vi "ODE-VI-28032016.vi"(0 "Param_Value":dbl[](array[numeric])=[0.35, 180.0, 0.3], 1 "Mod_Value":dbl[](array[numeric]), 3 "Param_IDs":string[](array[string])=["k1", "k2", "compartment"], 4 "Mod_IDs":string[](array[string]), 5 "Initial Conditions for  variables":dbl[](array[numeric])=[0.00015, 0.0], 6 "Simulation Parameters":T2={"Initial Time"=0.1, "Final Time"=1e-07, "Time Step"=0.0001, "Absolute Tolerance"=0.0, "Relative Tolerance"=1.0, "Type of Continuous Solver"=enum."Runge-Kutta 1 (Euler)", "Discrete Time Step"=1.0, "Minimum Time Step"=0.1, "Maximum Time Step"=0.0, "Initial Time Step"=10.0} {"Initial Time Step" min=0.0; "Maximum Time Step" min=0.0; "Minimum Time Step" min=0.0; "Discrete Time Step" min=0.0; "Relative Tolerance" min=0.0; "Absolute Tolerance" min=0.0; "Time Step" min=0.0}, 7 "ODE Right Hand Side":string[](array[string])=["-(compartment*k1*a0)+(compartment*k2*a1^2)", "-2*(compartment*k2*a1^2)+2*(compartment*k1*a0)"], 8 "Rest_Sp_IDs":string[](array[string]), 9 "Del Events":bool, 10 "Event Info":T1, 11 "X (name of variables)":string[](array[string])=["a0", "a1"], 12 "All Variables":string[](array[string]), 13 "Rest_Sp_Init_Amnt":string[](array[string])) -> (14 "Concentration vs. Time":cluster{"times":dbl[], dbl[]}[](graph), 16 "Mod_IDs Out":string[](array[string]), 17 "Rest_Sp_IDs Out":string[](array[string]), 19 "Sim Data":cluster{"times":dbl[], "outputs":dbl[][]} {"outputs" format="%#.9g"})   [LabVIEW 2014]
doc: "This example demonstrates how to use the polymorphic ODE solver in both Formula Sting mode and VI mode. Note that VI mode allows the user to set the values of constants via front panel controls, and the formula is implemented as a call by reference to another VI."
uses:
  ODE Simulation Parameters.ctl
  <vilib>/Simulation/Implementation/Shared/SIM Continuous Solvers.ctl
  Event Info.ctl
  Stop ODE.vi
  <vilib>/gmath/ode.llb/ODE Solver formula string.vi
  Sim status.vi
  <vilib>/gmath/NI_Gmath.lvlib
panel:
  out "error out":errorcluster
  out "subarray 2":dbl[](array[numeric])
  out "Array":dbl[][](array[numeric])
  out "transposed array":dbl[][](array[numeric])
  out "Assign Val":string[][](array[string])
  out "Assign Var Idx":i32[][](array[numeric])
  out "Var Idx":i32[](array[numeric])
  out "Math Val":string[](array[string])
  out "Math Op":string[](array[string])
  out "outputs":dbl[][](array[numeric])
  out "subarray":dbl[][](array[numeric])
  out "Flag":i32[](array[numeric])
  out "Delay Val Tot":dbl[](array[numeric])
  out "Delay Val":dbl[](array[numeric])
  out "Delay Val":dbl
  out "Priority":dbl[](array[numeric])
  out "Event Idx":i32
  out "Delay":dbl[](array[numeric])
  out "Total Mods":i32
  out "Time":dbl[](array[numeric])
  out "current data size":i32[](array[numeric])
  # "%"
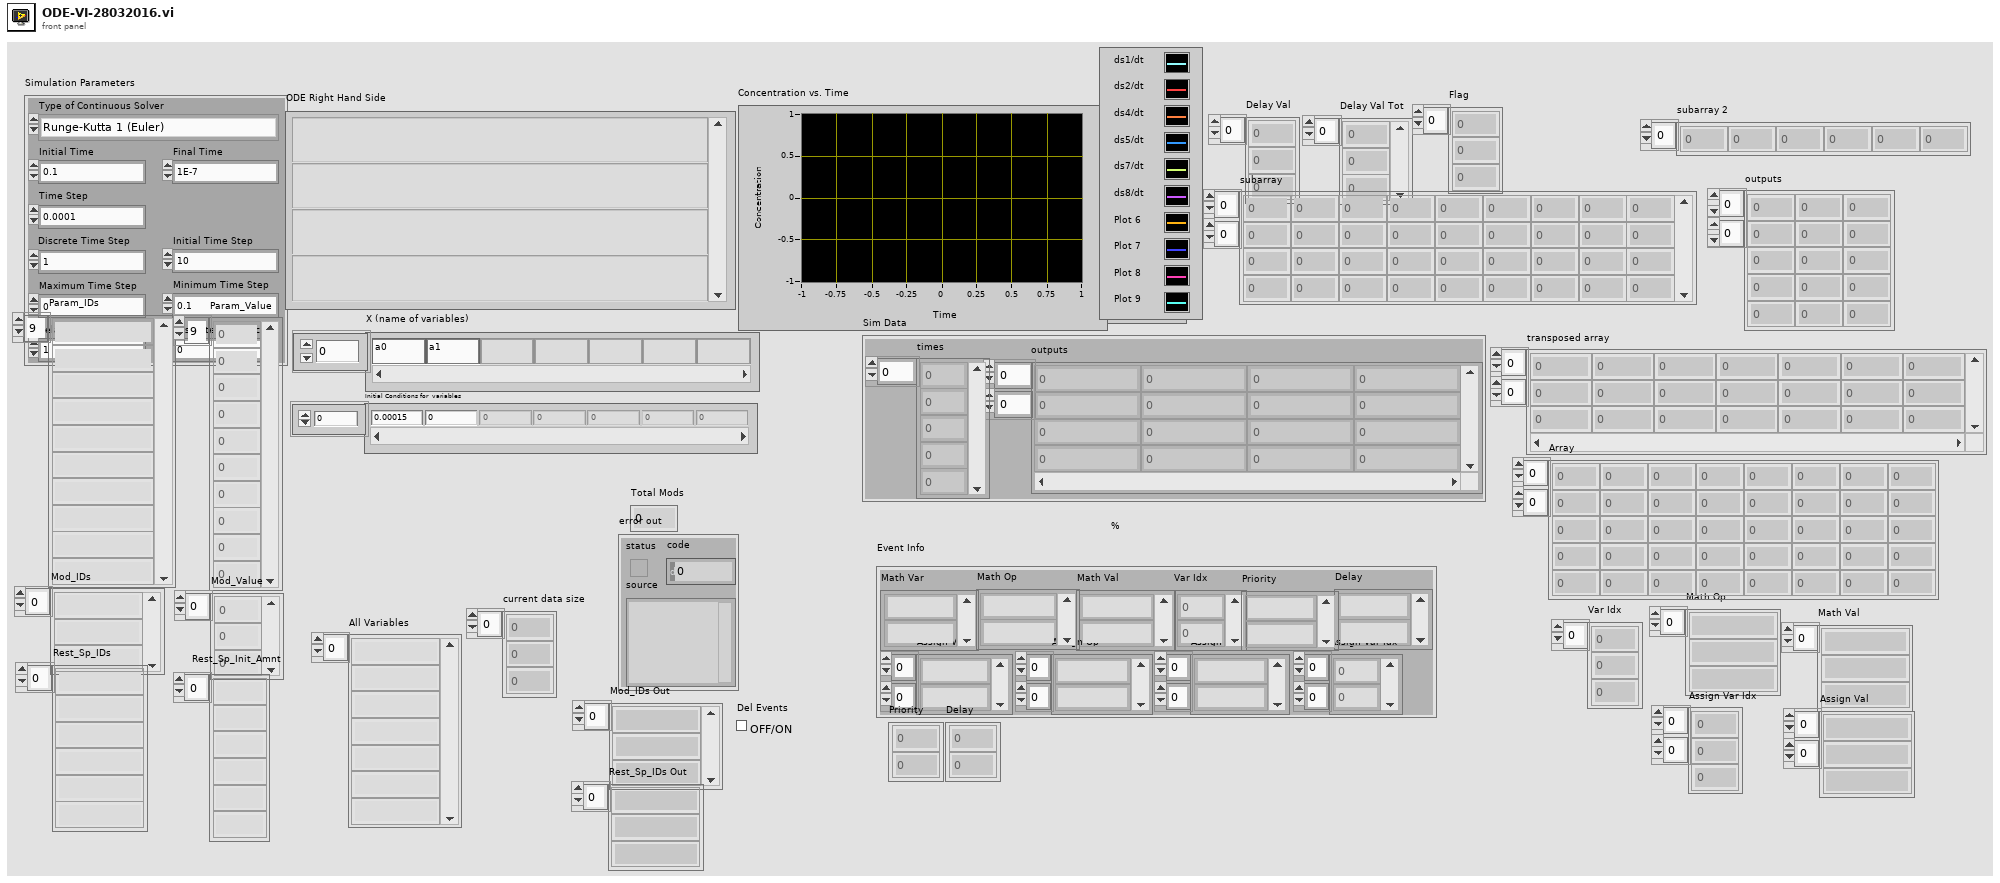
[diagram p1: front panel]
types:
  T1 = typedef "Event Info.ctl" = cluster{"Math Var":string[], "Math Op":string[], "Math Val":string[], "Assign Var":string[][], "Assign Op":string[][], "Assign Val":string[][], "Var Idx":i32[], "Assign Var Idx":i32[][], "Delay":string[], "Priority":string[]}
  T2 = typedef "ODE Simulation Parameters.ctl" = cluster{"Initial Time":dbl, "Final Time":dbl, "Time Step":dbl, "Absolute Tolerance":dbl, "Relative Tolerance":dbl, "Type of Continuous Solver":T3, "Discrete Time Step":dbl, "Minimum Time Step":dbl, "Maximum Time Step":dbl, "Initial Time Step":dbl}
  T3 = typedef "SIM Continuous Solvers.ctl" = enum16{"Runge-Kutta 1 (Euler)", "Runge-Kutta 2", "Runge-Kutta 3", "Runge-Kutta 4", "Runge-Kutta 23 (variable)", "Runge-Kutta 45 (variable)", "BDF (variable)", "Adams-Moulton (variable)", "Rosenbrock (variable)", "Discrete States Only"}
  T4 = cluster{"ODE Right Hand Side":string[], "X (name of variables)":string[], "time":string}
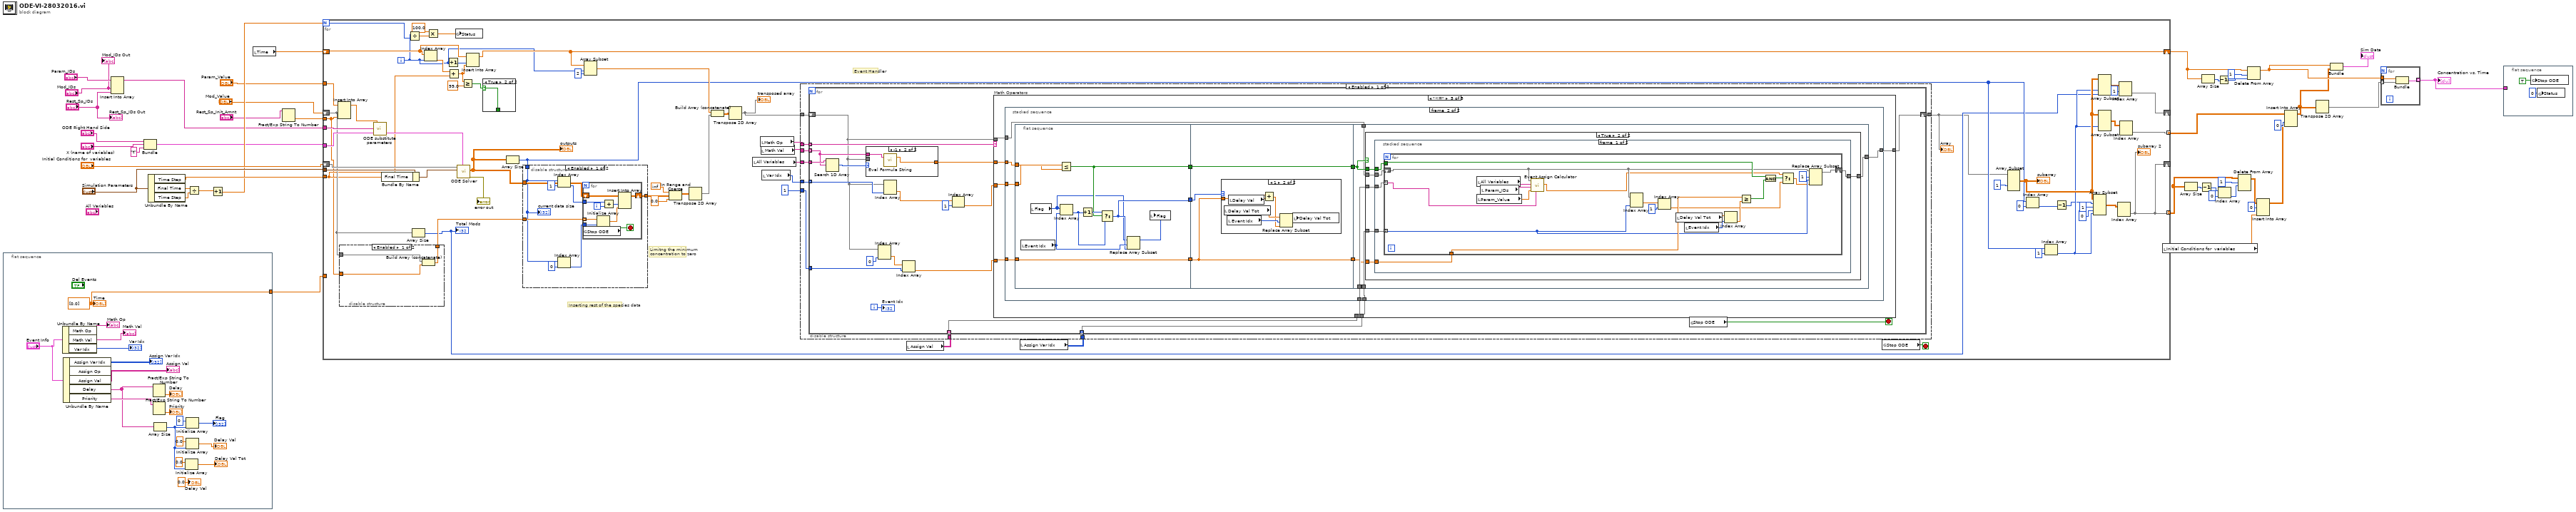
[diagram p0: block diagram]
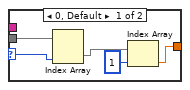
[diagram p5: hidden frame]
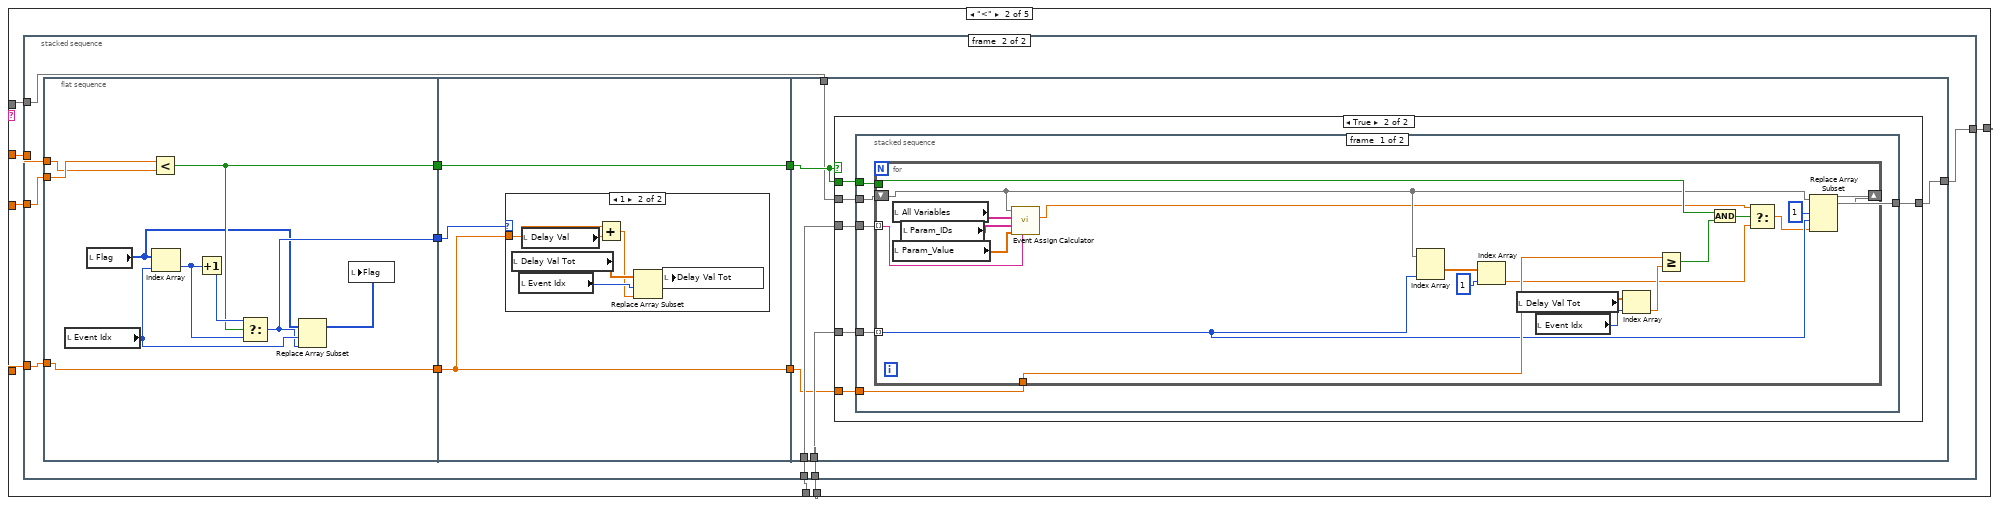
[diagram p7: hidden frame]
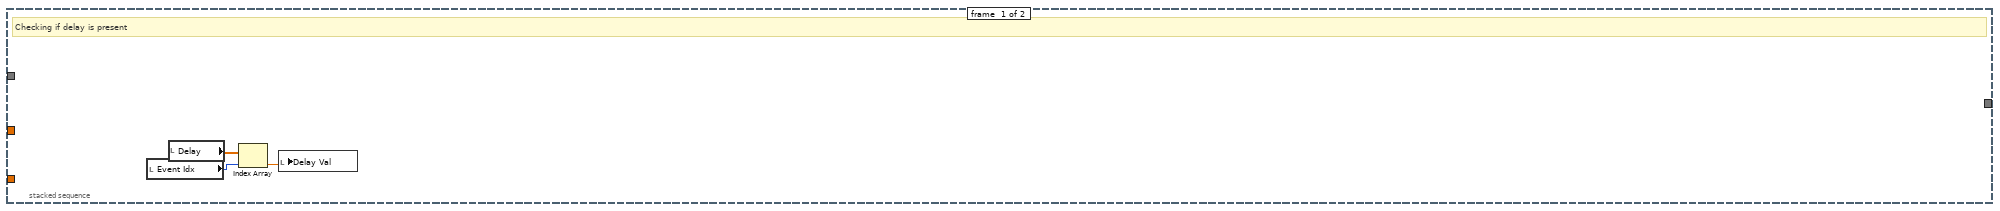
[diagram p8: hidden frame]
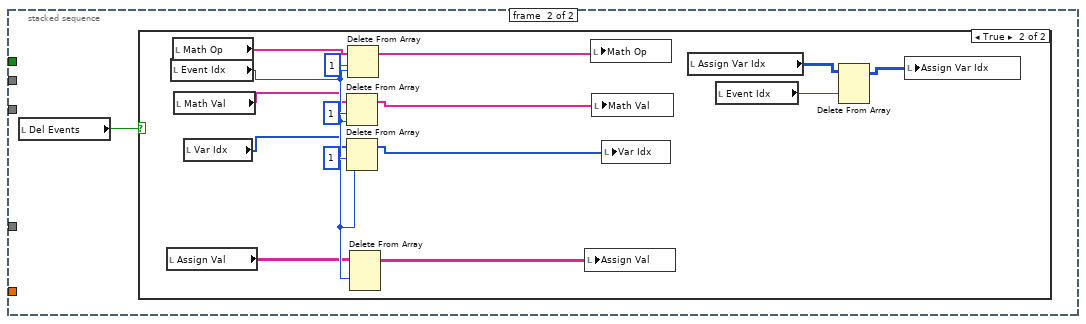
[diagram p11: hidden frame]
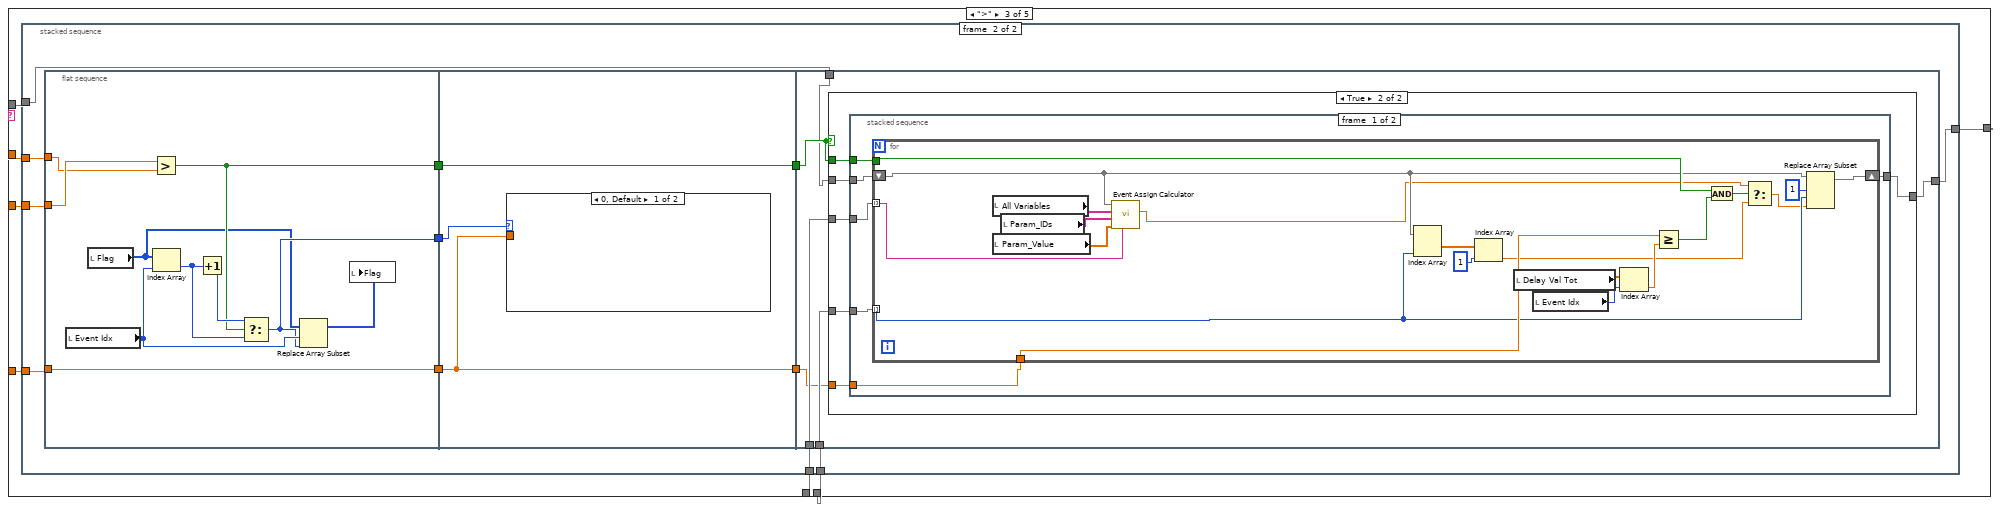
[diagram p13: hidden frame]
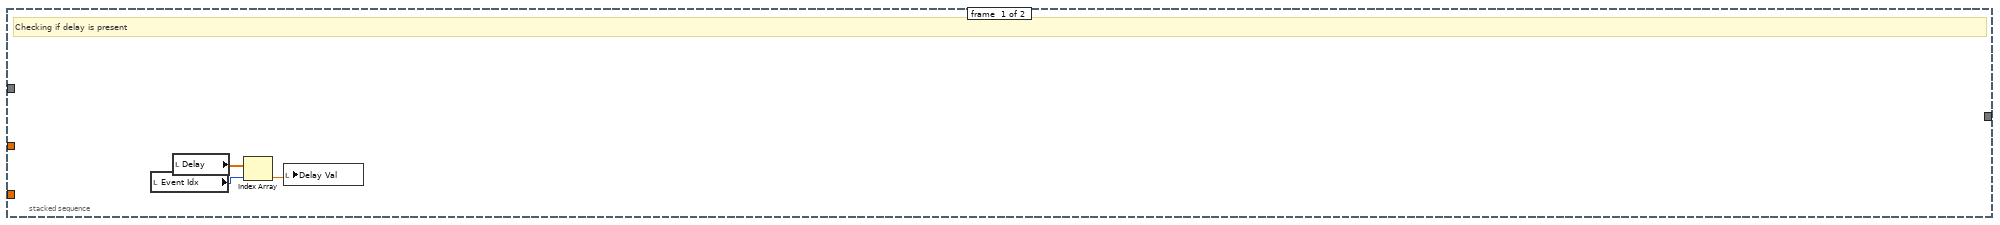
[diagram p14: hidden frame]
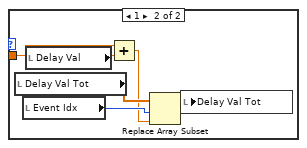
[diagram p15: hidden frame]
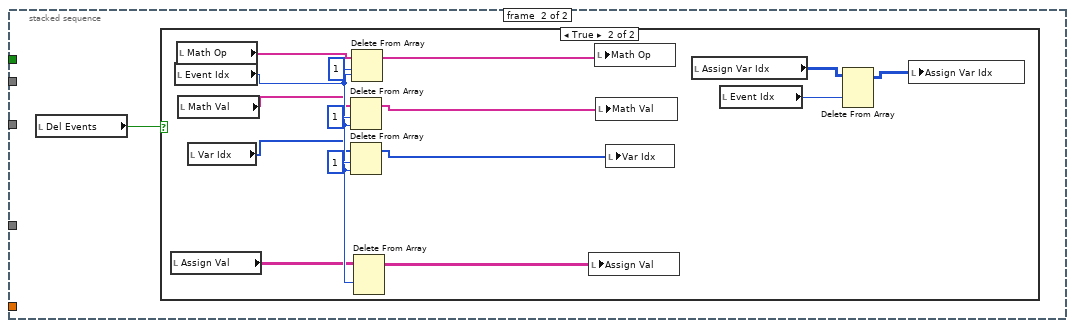
[diagram p17: hidden frame]
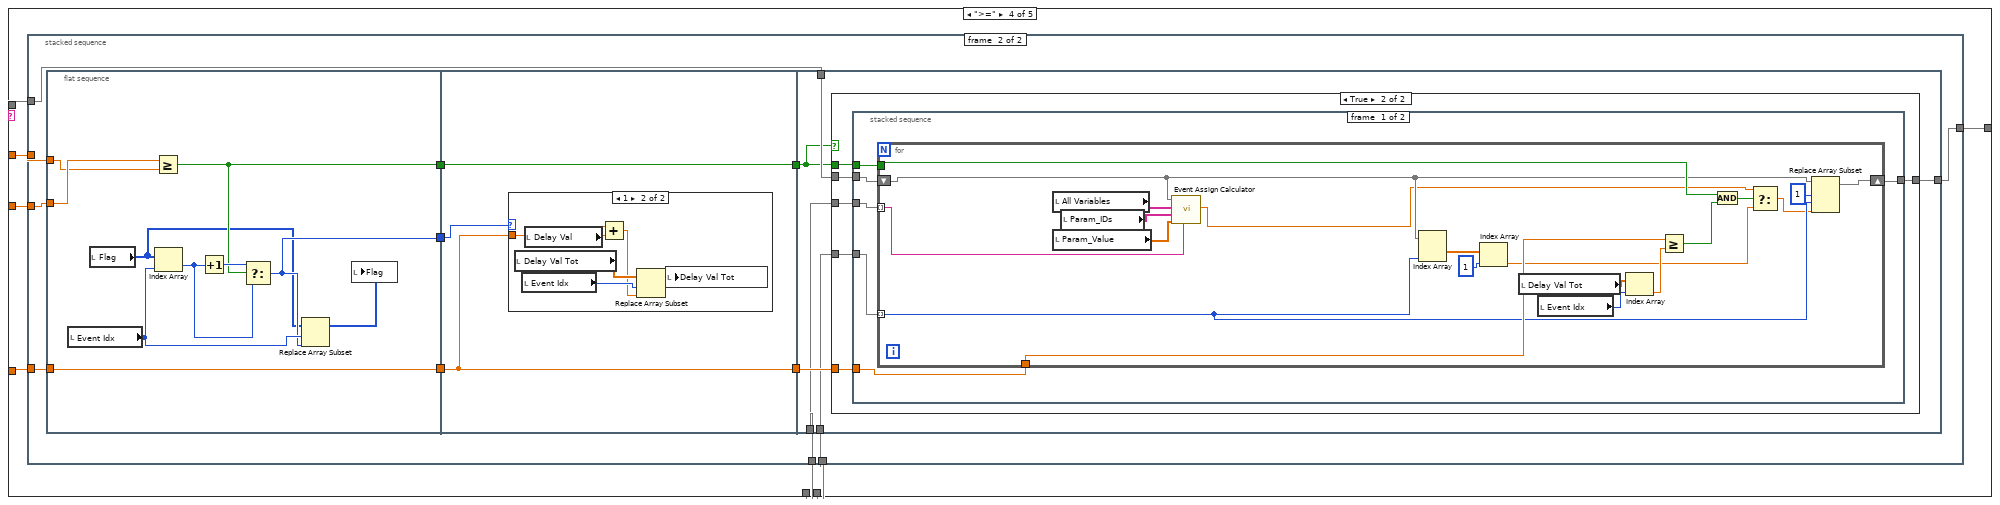
[diagram p19: hidden frame]
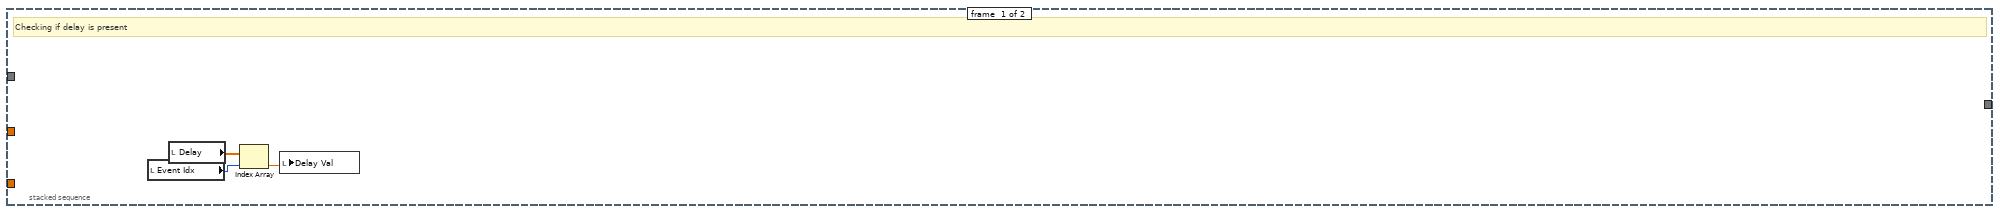
[diagram p20: hidden frame]
diagram:
  n1 = flat-sequence {
    tunnel: [w43] -> w4
    frame #0 {
      w43 = dbl[] [0.0]
      n2 = Unbundle By Name("Event Info") -> ("Math Op"=→"Math Op":string[], "Math Val"=→"Math Val":string[], "Var Idx"=→"Var Idx":i32[])
      n3 = Unbundle By Name("Event Info") -> ("Assign Var Idx"=→"Assign Var Idx":i32[][], "Assign Val"=→"Assign Val":string[][], "Delay"=w52:string[], "Priority"=w55:string[])  [unwired: 1 out]
      n4 = Fract/Exp String To Number(string=w52) -> (number=→"Delay":dbl[])  [unwired: 3 in, 1 out]
      n5 = Fract/Exp String To Number(string=w55) -> (number=→"Priority":dbl[])  [unwired: 3 in, 1 out]
      n6 = Array Size(array=w52) -> (size(s)=w47:i32)
      n7 = Initialize Array(0.0 ("element"), w47) -> (→"Delay Val Tot":dbl[])
      n8 = Initialize Array(0 ("element"), w47) -> (→"Flag":i32[])
      n9 = Initialize Array(0.0 ("element"), w47) -> (→"Delay Val":dbl[])
      "Time" <- w43
      "Delay Val" <- 0.0 ("Delay Val")
    }
  }
  n10 = Insert Into Array(array="Param_IDs", new element #1="Mod_IDs", new element #2="Rest_Sp_IDs") -> (w8:string[])  [unwired: 1 in]
  n11 = Bundle("ODE Right Hand Side"="ODE Right Hand Side", "X (name of variables)"="X (name of variables)", "time"="t") -> (w9:T4)  [unwired: 1 in]
  n12 = Unbundle By Name("Simulation Parameters") -> ("Time Step"=w33:dbl, "Final Time"=w35:dbl, "Time Step"=w34:dbl)
  n13 = Divide(x=w35, y=w34) -> (x/y=w31:dbl)
  n14 = Increment(x=w31) -> (x+1=w30:dbl)
  n15 = local read "Time"() -> (w32:dbl[])
  n16 = Fract/Exp String To Number(string="Rest_Sp_Init_Amnt") -> (number=w1:dbl[])  [unwired: 3 in, 1 out]
  n17 = for {
    N: w30 -> [w77]
    tunnel: "Simulation Parameters" -> [w108]
    shift-right: [w67] -> _
    shift-left: "Initial Conditions for  variables" -> [w123]
    shift-right: [w106] -> w28
    shift-left: w32 -> [w110]
    tunnel: [w67] -> w12 mode=indexing
    tunnel: w33 -> [w87]
    tunnel: [w101] -> w13 mode=indexing
    tunnel: w9 -> [w99]
    tunnel: w8 -> [w98]
    tunnel: "Param_Value" -> [w97]
    shift-right: [w80] -> _
    shift-left: "Mod_Value" -> [w93]
    tunnel: w4 -> [_]
    tunnel: w1 -> [w62]
    i -> [w78]
    stop <- w91 stop-if-true
    # "Event Handler"
    # "Limitng the minimum \nconcentration to zero"
    # "Inserting rest of the species data"
    n18 = Insert Into Array(array=w97, new element #1=w93, new element #2=w62) -> (w96:dbl[])  [unwired: 1 in]
    n19 = disable-structure shown="Enabled" {
      disable-tunnel: [w126 _] -> w121
      disable-tunnel: w93 -> [w125 _]
      disable-tunnel: w62 -> [w124 _]
      frame Enabled {
        n20 = Build Array (concatenate)(w125, w124) -> (w126:dbl[])
      }
      frame Disabled {
      }
    }
    n21 = call "ODE substitute parameters.vi"("Formula String Parameters"=w99, "parameters"=w98, "values"=w96) -> ("Formula String Parameters with substitutions"=w100:T4)  [unwired: 2 out]
    n22 = Bundle By Name(cluster=w108, "Final Time"=w87) -> (w107:T2)
    n23 = Divide(x=w78, y=w77) -> (x/y=w76:dbl)
    n24 = Array Size(array=w93) -> (size(s)=w92:i32)
    "Total Mods" <- w92
    n25 = Index Array(array=w110, index=w78) -> (element=w111:dbl)
    n26 = Multiply(x=100.0, y=w76) -> (x*y=w74:dbl)
    n27 = Increment(x=w78) -> (x+1=w109:i32)
    n28 = Add(x=w111, y=w87) -> (x+y=w84:dbl)
    n29 = global write "Sim status.vi" "Status"(w74) -> ()
    n30 = call-poly <vilib>:"ODE Solver.vi"("ODE RHS"=w100, "simulation parameters"=w107, "x0"=w123) -> ("error out"=→"error out":errorcluster, "outputs"=w122:dbl[][])  [unwired: 3 in, 4 out]
    "outputs" <- w122
    n31 = Greater Or Equal?(x=w84, y=99.0) -> (x >= y?=w82:bool)
    n32 = Insert Into Array(array=w110, index=w109, new element=w84) -> (w106:dbl[])
    n33 = case shown="True" w82 {
      selector: w82 -> [w145 w146]
      tunnel: [w145 w146] -> _
      frame False {
      }
      frame True {
      }
    }
    n34 = Array Size(array=w122) -> (size(s)=w103:i32[])
    n35 = disable-structure shown="Enabled" {
      disable-tunnel: w122 -> [w130 w144]
      disable-tunnel: w121 -> [w129 _]
      disable-tunnel: [w128 w144] -> w118
      disable-tunnel: w103 -> [w127 _]
      frame Enabled {
        n36 = Index Array(array=w127, index=1) -> (element=w133:i32)
        n37 = Index Array(array=w127, index=0) -> (element=w131:i32)
        n38 = for {
          tunnel: w129 -> [w140] mode=indexing
          tunnel: w133 -> [w142]
          tunnel: w131 -> [w139]
          shift-right: [w136] -> w128
          shift-left: w130 -> [w137]
          i -> [w143]
          stop <- w135 stop-if-true
          n39 = global read "Stop ODE.vi" "Stop ODE"() -> (w135:bool)
          n40 = Initialize Array(w140, w139) -> (w138:dbl[])
          n41 = Add(x=w142, y=w143) -> (x+y=w141:i32)
          n42 = Insert Into Array(array=w137, index (col)=w141, new element=w138) -> (w136:dbl[][])  [unwired: 1 in]
        }
        "current data size" <- w127
      }
      frame Disabled {
      }
    }
    n43 = Array Subset(array=w106, index=w78, length=2) -> (w104:dbl[])
    n44 = In Range and Coerce(upper limit=inf, x=w118, lower limit=0.0) -> (coerced(x)=w89:dbl[][])  [unwired: 1 out]
    n45 = Transpose 2D Array(2D array=w89) -> (transposed array=w88:dbl[][])
    n46 = Build Array (concatenate)(w104, w88) -> (w90:dbl[][])
    n47 = Transpose 2D Array(2D array=w90) -> (transposed array=w86:dbl[][])
    "transposed array" <- w86
    n48 = local read "All Variables"() -> (w68:string[])
    n49 = local read "Math Op"() -> (w73:string[])
    n50 = local read "Math Val"() -> (w72:string[])
    n51 = local read "Var Idx"() -> (w71:i32[])
    n52 = local read "Assign Val"() -> (w69:string[][])
    n53 = local read "Assign Var Idx"() -> (w70:i32[][])
    n54 = disable-structure shown="Enabled" {
      disable-tunnel: w73 -> [w155 w576]
      disable-tunnel: w72 -> [w154 w577]
      disable-tunnel: w71 -> [w153 w578]
      disable-tunnel: w69 -> [w148 w575]
      disable-tunnel: w70 -> [w152 w574]
      disable-tunnel: [w151 w580] -> w66
      disable-tunnel: w86 -> [w150 w581]
      disable-tunnel: 1 ("index") -> [w149 w579]
      disable-tunnel: w68 -> [w147 _]
      frame Enabled {
        n55 = for {
          tunnel: w155 -> [w174] mode=indexing
          tunnel: w154 -> [w158] mode=indexing
          tunnel: w153 -> [w173] mode=indexing
          tunnel: w148 -> [w169] mode=indexing
          tunnel: w152 -> [w172] mode=indexing
          shift-right: [w167] -> w151
          shift-left: w150 -> [w156]
          tunnel: w149 -> [w161]
          tunnel: w147 -> [w159]
          i -> [w170]
          stop <- w171 stop-if-true
          n56 = Search 1D Array(1D array=w159, element=w158) -> (index of element=w157:i32)  [unwired: 1 in]
          n57 = case shown="-1" w157 {
            selector: w157 -> [w178 _]
            tunnel: [w175 w180] -> w168
            tunnel: w158 -> [_ w181]
            tunnel: w156 -> [w179 _]
            frame 0, Default {
              n58 = Index Array(array=w179, index (col)=w178) -> (element=w176:dbl[])  [unwired: 1 in]
              n59 = Index Array(array=w176, index=1) -> (element=w175:dbl)
            }
            frame -1 {
              n60 = call <vilib>:"Eval Formula String.vi"("formula"=w181) -> ("y value"=w180:dbl)  [unwired: 1 in, 1 out]
            }
          }
          n61 = Index Array(array=w156, index (col)=0 ("disabled index (col)")) -> (element=w162:dbl[])  [unwired: 1 in]
          n62 = Index Array(array=w156, index (col)=w173) -> (element=w165:dbl[])  [unwired: 1 in]
          n63 = Index Array(array=w162, index=w161) -> (element=w160:dbl)
          n64 = Index Array(array=w165, index=1) -> (element=w164:dbl)
          n65 = case "Math Operators" shown="\"<=\"" w174 {
            tunnel: w168 -> [_ w188 w284 w380 w476]
            tunnel: [w182 w187 w283 w379 w475] -> w167
            tunnel: w156 -> [w182 w189 w285 w381 w477]
            tunnel: w169 -> [_ w186 w282 w378 w474]
            tunnel: w172 -> [_ w185 w281 w377 w473]
            tunnel: w164 -> [_ w184 w280 w375 w472]
            tunnel: w160 -> [_ w183 w279 w376 w471]
            frame "False", Default {
            }
            frame "<" {
              n66 = stacked-sequence {
                tunnel: w188 -> [_ w204]
                tunnel: w189 -> [_ w196]
                tunnel: [_ w195] -> w187
                tunnel: w186 -> [_ w198]
                tunnel: w185 -> [_ w197]
                tunnel: w184 -> [_ w194]
                tunnel: w183 -> [_ w193]
                frame #0 {
                  # "Checking if delay is present"
                  n67 = local read "Event Idx"() -> (w191:i32)
                  n68 = local read "Delay"() -> (w192:dbl[])
                  n69 = Index Array(array=w192, index=w191) -> (element=w190:dbl)
                  n70 = local write "Delay Val"(w190) -> ()
                }
                frame #1 {
                  n71 = flat-sequence {
                    tunnel: w194 -> [w214]
                    tunnel: w204 -> [w213]
                    tunnel: [w208] -> w203
                    tunnel: [w207] -> w202
                    tunnel: [w205] -> w201
                    tunnel: w193 -> [w205]
                    tunnel: w203 -> [w216]
                    tunnel: w202 -> [w217]
                    tunnel: w201 -> [w215]
                    tunnel: [w217] -> w200
                    tunnel: [w215] -> w199
                    tunnel: w200 -> [w229]
                    tunnel: w199 -> [w225]
                    tunnel: w196 -> [w228]
                    tunnel: w197 -> [w226]
                    tunnel: w198 -> [w227]
                    tunnel: [w224] -> w195
                    frame #0 {
                      n72 = local read "Event Idx"() -> (w211:i32)
                      n73 = local read "Flag"() -> (w206:i32[])
                      n74 = Less?(x=w214, y=w213) -> (x < y?=w207:bool)
                      n75 = Index Array(array=w206, index=w211) -> (element=w210:i32)
                      n76 = Increment(x=w210) -> (x+1=w209:i32)
                      n77 = Select(t=w209, s=w207, f=w210) -> (s? t:f=w208:i32)
                      n78 = Replace Array Subset(array=w206, new element=w208, index=w211) -> (w212:i32[])
                      n79 = local write "Flag"(w212) -> ()
                    }
                    frame #1 {
                      n80 = case shown="1" w216 {
                        tunnel: w215 -> [_ w222]
                        frame 0, Default {
                        }
                        frame 1 {
                          n81 = local read "Delay Val Tot"() -> (w221:dbl[])
                          n82 = local read "Event Idx"() -> (w219:i32)
                          n83 = local read "Delay Val"() -> (w223:dbl)
                          n84 = Add(x=w222, y=w223) -> (x+y=w218:dbl)
                          n85 = Replace Array Subset(array=w221, new element=w218, index=w219) -> (w220:dbl[])
                          n86 = local write "Delay Val Tot"(w220) -> ()
                        }
                      }
                    }
                    frame #2 {
                      n87 = case shown="True" w229 {
                        tunnel: w229 -> [_ w236]
                        tunnel: w225 -> [_ w235]
                        tunnel: w228 -> [w230 w234]
                        tunnel: w226 -> [_ w233]
                        tunnel: w227 -> [_ w232]
                        tunnel: [w230 w231] -> w224
                        frame False {
                        }
                        frame True {
                          n88 = stacked-sequence {
                            tunnel: w236 -> [w242 _]
                            tunnel: w235 -> [w241 _]
                            tunnel: w234 -> [w240 _]
                            tunnel: w233 -> [w239 _]
                            tunnel: w232 -> [w238 _]
                            tunnel: [w237 _] -> w231
                            frame #0 {
                              n89 = for {
                                tunnel: w242 -> [w260]
                                tunnel: w241 -> [w259]
                                tunnel: w239 -> [w251] mode=indexing
                                tunnel: w238 -> [w244] mode=indexing
                                shift-right: [w249] -> w237
                                shift-left: w240 -> [w248]
                                n90 = local read "All Variables"() -> (w247:string[])
                                n91 = local read "Param_Value"() -> (w245:dbl[])
                                n92 = local read "Param_IDs"() -> (w246:string[])
                                n93 = call "Event Assign Calculator.vi"("Assign Val"=w244, "Param_Value"=w245, "Param_IDs"=w246, "All Variables"=w247, "transposed array"=w248) -> ("y value"=w243:dbl)  [unwired: 6 in]
                                n94 = Index Array(array=w248, index (col)=w251) -> (element=w254:dbl[])  [unwired: 1 in]
                                n95 = Index Array(array=w254, index=1) -> (element=w253:dbl)
                                n96 = local read "Delay Val Tot"() -> (w258:dbl[])
                                n97 = local read "Event Idx"() -> (w257:i32)
                                n98 = Index Array(array=w258, index=w257) -> (element=w256:dbl)
                                n99 = Greater Or Equal?(x=w259, y=w256) -> (x >= y?=w261:bool)
                                n100 = And(x=w260, y=w261) -> (x .and. y?=w262:bool)
                                n101 = Select(t=w243, s=w262, f=w253) -> (s? t:f=w250:dbl)
                                n102 = Replace Array Subset(array=w248, new element=w250, index (row)=1, index (col)=w251) -> (w249:dbl[][])
                              }
                            }
                            frame #1 {
                              n103 = local read "Del Events"() -> (w263:bool)
                              n104 = case shown="True" w263 {
                                frame False {
                                }
                                frame True {
                                n105 = local read "Assign Val"() -> (w268:string[][])
                                n106 = local read "Event Idx"() -> (w275:i32)
                                n107 = local read "Math Op"() -> (w274:string[])
                                n108 = local read "Math Val"() -> (w273:string[])
                                n109 = local read "Var Idx"() -> (w272:i32[])
                                n110 = Delete From Array(array=w273, length=1, index=w275) -> (array with subset deleted=w270:string[])  [unwired: 1 out]
                                n111 = Delete From Array(array=w272, length=1, index=w275) -> (array with subset deleted=w269:i32[])  [unwired: 1 out]
                                n112 = Delete From Array(array=w274, length=1, index=w275) -> (array with subset deleted=w271:string[])  [unwired: 1 out]
                                n113 = Delete From Array(array=w268, index (row)=w275) -> (array with subset deleted=w267:string[][])  [unwired: 2 in, 1 out]
                                n114 = local write "Assign Val"(w267) -> ()
                                n115 = local write "Math Op"(w271) -> ()
                                n116 = local write "Math Val"(w270) -> ()
                                n117 = local write "Var Idx"(w269) -> ()
                                n118 = local read "Assign Var Idx"() -> (w266:i32[][])
                                n119 = local read "Event Idx"() -> (w265:i32)
                                n120 = Delete From Array(array=w266, index (row)=w265) -> (array with subset deleted=w264:i32[][])  [unwired: 2 in, 1 out]
                                n121 = local write "Assign Var Idx"(w264) -> ()
                                }
                              }
                            }
                          }
                        }
                      }
                    }
                  }
                }
              }
            }
            frame ">" {
              n122 = stacked-sequence {
                tunnel: w284 -> [_ w300]
                tunnel: w285 -> [_ w292]
                tunnel: [_ w291] -> w283
                tunnel: w282 -> [_ w294]
                tunnel: w281 -> [_ w293]
                tunnel: w280 -> [_ w290]
                tunnel: w279 -> [_ w289]
                frame #0 {
                  # "Checking if delay is present"
                  n123 = local read "Event Idx"() -> (w287:i32)
                  n124 = local read "Delay"() -> (w288:dbl[])
                  n125 = Index Array(array=w288, index=w287) -> (element=w286:dbl)
                  n126 = local write "Delay Val"(w286) -> ()
                }
                frame #1 {
                  n127 = flat-sequence {
                    tunnel: w290 -> [w310]
                    tunnel: w300 -> [w309]
                    tunnel: w289 -> [w308]
                    tunnel: [w303] -> w299
                    tunnel: [w302] -> w298
                    tunnel: [w308] -> w297
                    tunnel: w299 -> [w312]
                    tunnel: w298 -> [w313]
                    tunnel: w297 -> [w311]
                    tunnel: [w313] -> w296
                    tunnel: [w311] -> w295
                    tunnel: w296 -> [w325]
                    tunnel: w295 -> [w321]
                    tunnel: w292 -> [w324]
                    tunnel: w293 -> [w322]
                    tunnel: w294 -> [w323]
                    tunnel: [w320] -> w291
                    frame #0 {
                      n128 = local read "Event Idx"() -> (w306:i32)
                      n129 = local read "Flag"() -> (w301:i32[])
                      n130 = Greater?(x=w310, y=w309) -> (0:w302:bool)
                      n131 = Index Array(array=w301, index=w306) -> (element=w305:i32)
                      n132 = Increment(x=w305) -> (x+1=w304:i32)
                      n133 = Select(t=w304, s=w302, f=w305) -> (s? t:f=w303:i32)
                      n134 = Replace Array Subset(array=w301, new element=w303, index=w306) -> (w307:i32[])
                      n135 = local write "Flag"(w307) -> ()
                    }
                    frame #1 {
                      n136 = case shown="0, Default" w312 {
                        tunnel: w311 -> [_ w318]
                        frame 0, Default {
                        }
                        frame 1 {
                          n137 = local read "Delay Val Tot"() -> (w317:dbl[])
                          n138 = local read "Event Idx"() -> (w315:i32)
                          n139 = local read "Delay Val"() -> (w319:dbl)
                          n140 = Add(x=w318, y=w319) -> (x+y=w314:dbl)
                          n141 = Replace Array Subset(array=w317, new element=w314, index=w315) -> (w316:dbl[])
                          n142 = local write "Delay Val Tot"(w316) -> ()
                        }
                      }
                    }
                    frame #2 {
                      n143 = case shown="True" w325 {
                        tunnel: w325 -> [_ w332]
                        tunnel: w321 -> [_ w331]
                        tunnel: w324 -> [w326 w330]
                        tunnel: w322 -> [_ w329]
                        tunnel: w323 -> [_ w328]
                        tunnel: [w326 w327] -> w320
                        frame False {
                        }
                        frame True {
                          n144 = stacked-sequence {
                            tunnel: w332 -> [w336 _]
                            tunnel: w331 -> [w333 _]
                            tunnel: w330 -> [w335 _]
                            tunnel: w329 -> [w337 _]
                            tunnel: w328 -> [w334 _]
                            tunnel: [w338 _] -> w327
                            frame #0 {
                              n145 = for {
                                tunnel: w336 -> [w356]
                                tunnel: w333 -> [w355]
                                tunnel: w337 -> [w347] mode=indexing
                                tunnel: w334 -> [w341] mode=indexing
                                shift-right: [w345] -> w338
                                shift-left: w335 -> [w340]
                                n146 = local read "All Variables"() -> (w344:string[])
                                n147 = local read "Param_Value"() -> (w342:dbl[])
                                n148 = local read "Param_IDs"() -> (w343:string[])
                                n149 = call "Event Assign Calculator.vi"("Assign Val"=w341, "Param_Value"=w342, "Param_IDs"=w343, "All Variables"=w344, "transposed array"=w340) -> ("y value"=w339:dbl)  [unwired: 6 in]
                                n150 = Index Array(array=w340, index (col)=w347) -> (element=w350:dbl[])  [unwired: 1 in]
                                n151 = Index Array(array=w350, index=1) -> (element=w349:dbl)
                                n152 = local read "Delay Val Tot"() -> (w354:dbl[])
                                n153 = local read "Event Idx"() -> (w353:i32)
                                n154 = Index Array(array=w354, index=w353) -> (element=w352:dbl)
                                n155 = Greater Or Equal?(x=w355, y=w352) -> (x >= y?=w357:bool)
                                n156 = And(x=w356, y=w357) -> (x .and. y?=w358:bool)
                                n157 = Select(t=w339, s=w358, f=w349) -> (s? t:f=w346:dbl)
                                n158 = Replace Array Subset(array=w340, new element=w346, index (row)=1, index (col)=w347) -> (w345:dbl[][])
                              }
                            }
                            frame #1 {
                              n159 = local read "Del Events"() -> (w359:bool)
                              n160 = case shown="True" w359 {
                                frame False {
                                }
                                frame True {
                                n161 = local read "Assign Val"() -> (w364:string[][])
                                n162 = local read "Event Idx"() -> (w371:i32)
                                n163 = local read "Math Op"() -> (w370:string[])
                                n164 = local read "Math Val"() -> (w369:string[])
                                n165 = local read "Var Idx"() -> (w368:i32[])
                                n166 = Delete From Array(array=w369, length=1, index=w371) -> (array with subset deleted=w366:string[])  [unwired: 1 out]
                                n167 = Delete From Array(array=w368, length=1, index=w371) -> (array with subset deleted=w365:i32[])  [unwired: 1 out]
                                n168 = Delete From Array(array=w370, length=1, index=w371) -> (array with subset deleted=w367:string[])  [unwired: 1 out]
                                n169 = Delete From Array(array=w364, index (row)=w371) -> (array with subset deleted=w363:string[][])  [unwired: 2 in, 1 out]
                                n170 = local write "Assign Val"(w363) -> ()
                                n171 = local write "Math Op"(w367) -> ()
                                n172 = local write "Math Val"(w366) -> ()
                                n173 = local write "Var Idx"(w365) -> ()
                                n174 = local read "Assign Var Idx"() -> (w362:i32[][])
                                n175 = local read "Event Idx"() -> (w361:i32)
                                n176 = Delete From Array(array=w362, index (row)=w361) -> (array with subset deleted=w360:i32[][])  [unwired: 2 in, 1 out]
                                n177 = local write "Assign Var Idx"(w360) -> ()
                                }
                              }
                            }
                          }
                        }
                      }
                    }
                  }
                }
              }
            }
            frame ">=" {
              n178 = stacked-sequence {
                tunnel: w380 -> [_ w396]
                tunnel: w381 -> [_ w388]
                tunnel: [_ w387] -> w379
                tunnel: w378 -> [_ w390]
                tunnel: w377 -> [_ w389]
                tunnel: w376 -> [_ w386]
                tunnel: w375 -> [_ w385]
                frame #0 {
                  # "Checking if delay is present"
                  n179 = local read "Event Idx"() -> (w383:i32)
                  n180 = local read "Delay"() -> (w384:dbl[])
                  n181 = Index Array(array=w384, index=w383) -> (element=w382:dbl)
                  n182 = local write "Delay Val"(w382) -> ()
                }
                frame #1 {
                  n183 = flat-sequence {
                    tunnel: w385 -> [w406]
                    tunnel: w396 -> [w405]
                    tunnel: w386 -> [w404]
                    tunnel: [w399] -> w395
                    tunnel: [w398] -> w394
                    tunnel: [w404] -> w393
                    tunnel: w395 -> [w408]
                    tunnel: w394 -> [w409]
                    tunnel: w393 -> [w407]
                    tunnel: [w409] -> w392
                    tunnel: [w407] -> w391
                    tunnel: w392 -> [w416]
                    tunnel: w391 -> [w421]
                    tunnel: w388 -> [w420]
                    tunnel: w389 -> [w419]
                    tunnel: w390 -> [w418]
                    tunnel: [w417] -> w387
                    frame #0 {
                      n184 = local read "Event Idx"() -> (w402:i32)
                      n185 = local read "Flag"() -> (w397:i32[])
                      n186 = Greater Or Equal?(x=w406, y=w405) -> (x >= y?=w398:bool)
                      n187 = Index Array(array=w397, index=w402) -> (element=w401:i32)
                      n188 = Increment(x=w401) -> (x+1=w400:i32)
                      n189 = Select(t=w400, s=w398, f=w401) -> (s? t:f=w399:i32)
                      n190 = Replace Array Subset(array=w397, new element=w399, index=w402) -> (w403:i32[])
                      n191 = local write "Flag"(w403) -> ()
                    }
                    frame #1 {
                      n192 = case shown="1" w408 {
                        tunnel: w407 -> [_ w414]
                        frame 0, Default {
                        }
                        frame 1 {
                          n193 = local read "Delay Val Tot"() -> (w413:dbl[])
                          n194 = local read "Event Idx"() -> (w411:i32)
                          n195 = local read "Delay Val"() -> (w415:dbl)
                          n196 = Add(x=w414, y=w415) -> (x+y=w410:dbl)
                          n197 = Replace Array Subset(array=w413, new element=w410, index=w411) -> (w412:dbl[])
                          n198 = local write "Delay Val Tot"(w412) -> ()
                        }
                      }
                    }
                    frame #2 {
                      n199 = case shown="True" w416 {
                        tunnel: w416 -> [_ w428]
                        tunnel: w421 -> [_ w427]
                        tunnel: w420 -> [w422 w426]
                        tunnel: w419 -> [_ w425]
                        tunnel: w418 -> [_ w424]
                        tunnel: [w422 w423] -> w417
                        frame False {
                        }
                        frame True {
                          n200 = stacked-sequence {
                            tunnel: w428 -> [w433 _]
                            tunnel: w427 -> [w430 _]
                            tunnel: w426 -> [w434 _]
                            tunnel: w425 -> [w431 _]
                            tunnel: w424 -> [w432 _]
                            tunnel: [w429 _] -> w423
                            frame #0 {
                              n201 = for {
                                tunnel: w433 -> [w452]
                                tunnel: w430 -> [w451]
                                tunnel: w431 -> [w443] mode=indexing
                                tunnel: w432 -> [w437] mode=indexing
                                shift-right: [w441] -> w429
                                shift-left: w434 -> [w436]
                                n202 = local read "All Variables"() -> (w440:string[])
                                n203 = local read "Param_Value"() -> (w438:dbl[])
                                n204 = local read "Param_IDs"() -> (w439:string[])
                                n205 = call "Event Assign Calculator.vi"("Assign Val"=w437, "Param_Value"=w438, "Param_IDs"=w439, "All Variables"=w440, "transposed array"=w436) -> ("y value"=w435:dbl)  [unwired: 6 in]
                                n206 = Index Array(array=w436, index (col)=w443) -> (element=w446:dbl[])  [unwired: 1 in]
                                n207 = Index Array(array=w446, index=1) -> (element=w445:dbl)
                                n208 = local read "Delay Val Tot"() -> (w450:dbl[])
                                n209 = local read "Event Idx"() -> (w449:i32)
                                n210 = Index Array(array=w450, index=w449) -> (element=w448:dbl)
                                n211 = Greater Or Equal?(x=w451, y=w448) -> (x >= y?=w453:bool)
                                n212 = And(x=w452, y=w453) -> (x .and. y?=w454:bool)
                                n213 = Select(t=w435, s=w454, f=w445) -> (s? t:f=w442:dbl)
                                n214 = Replace Array Subset(array=w436, new element=w442, index (row)=1, index (col)=w443) -> (w441:dbl[][])
                              }
                            }
                            frame #1 {
                              n215 = local read "Del Events"() -> (w455:bool)
                              n216 = case shown="True" w455 {
                                frame False {
                                }
                                frame True {
                                n217 = local read "Assign Val"() -> (w460:string[][])
                                n218 = local read "Event Idx"() -> (w467:i32)
                                n219 = local read "Math Op"() -> (w466:string[])
                                n220 = local read "Math Val"() -> (w465:string[])
                                n221 = local read "Var Idx"() -> (w464:i32[])
                                n222 = Delete From Array(array=w465, length=1, index=w467) -> (array with subset deleted=w462:string[])  [unwired: 1 out]
                                n223 = Delete From Array(array=w464, length=1, index=w467) -> (array with subset deleted=w461:i32[])  [unwired: 1 out]
                                n224 = Delete From Array(array=w466, length=1, index=w467) -> (array with subset deleted=w463:string[])  [unwired: 1 out]
                                n225 = Delete From Array(array=w460, index (row)=w467) -> (array with subset deleted=w459:string[][])  [unwired: 2 in, 1 out]
                                n226 = local write "Assign Val"(w459) -> ()
                                n227 = local write "Math Op"(w463) -> ()
                                n228 = local write "Math Val"(w462) -> ()
                                n229 = local write "Var Idx"(w461) -> ()
                                n230 = local read "Assign Var Idx"() -> (w458:i32[][])
                                n231 = local read "Event Idx"() -> (w457:i32)
                                n232 = Delete From Array(array=w458, index (row)=w457) -> (array with subset deleted=w456:i32[][])  [unwired: 2 in, 1 out]
                                n233 = local write "Assign Var Idx"(w456) -> ()
                                }
                              }
                            }
                          }
                        }
                      }
                    }
                  }
                }
              }
            }
            frame "<=" {
              n234 = stacked-sequence {
                tunnel: w476 -> [_ w492]
                tunnel: w477 -> [_ w484]
                tunnel: [_ w481] -> w475
                tunnel: w474 -> [_ w486]
                tunnel: w473 -> [_ w485]
                tunnel: w472 -> [_ w483]
                tunnel: w471 -> [_ w482]
                frame #0 {
                  # "Checking if delay is present"
                  n235 = local read "Event Idx"() -> (w479:i32)
                  n236 = local read "Delay"() -> (w480:dbl[])
                  n237 = Index Array(array=w480, index=w479) -> (element=w478:dbl)
                  n238 = local write "Delay Val"(w478) -> ()
                }
                frame #1 {
                  n239 = flat-sequence {
                    tunnel: w483 -> [w502]
                    tunnel: w492 -> [w501]
                    tunnel: w482 -> [w500]
                    tunnel: [w495] -> w491
                    tunnel: [w494] -> w490
                    tunnel: [w500] -> w489
                    tunnel: w491 -> [w504]
                    tunnel: w490 -> [w505]
                    tunnel: w489 -> [w503]
                    tunnel: [w505] -> w488
                    tunnel: [w503] -> w487
                    tunnel: w488 -> [w517]
                    tunnel: w487 -> [w513]
                    tunnel: w484 -> [w516]
                    tunnel: w485 -> [w514]
                    tunnel: w486 -> [w515]
                    tunnel: [w512] -> w481
                    frame #0 {
                      n240 = local read "Event Idx"() -> (w498:i32)
                      n241 = local read "Flag"() -> (w493:i32[])
                      n242 = Less Or Equal?(x=w502, y=w501) -> (x <= y?=w494:bool)
                      n243 = Index Array(array=w493, index=w498) -> (element=w497:i32)
                      n244 = Increment(x=w497) -> (x+1=w496:i32)
                      n245 = Select(t=w496, s=w494, f=w497) -> (s? t:f=w495:i32)
                      n246 = Replace Array Subset(array=w493, new element=w495, index=w498) -> (w499:i32[])
                      n247 = local write "Flag"(w499) -> ()
                    }
                    frame #1 {
                      n248 = case shown="1" w504 {
                        tunnel: w503 -> [_ w510]
                        frame 0, Default {
                        }
                        frame 1 {
                          n249 = local read "Delay Val Tot"() -> (w509:dbl[])
                          n250 = local read "Event Idx"() -> (w507:i32)
                          n251 = local read "Delay Val"() -> (w511:dbl)
                          n252 = Add(x=w510, y=w511) -> (x+y=w506:dbl)
                          n253 = Replace Array Subset(array=w509, new element=w506, index=w507) -> (w508:dbl[])
                          n254 = local write "Delay Val Tot"(w508) -> ()
                        }
                      }
                    }
                    frame #2 {
                      n255 = case shown="True" w517 {
                        tunnel: w517 -> [_ w524]
                        tunnel: w513 -> [_ w523]
                        tunnel: w516 -> [w518 w522]
                        tunnel: w514 -> [_ w521]
                        tunnel: w515 -> [_ w520]
                        tunnel: [w518 w519] -> w512
                        frame False {
                        }
                        frame True {
                          n256 = stacked-sequence {
                            tunnel: w524 -> [w530 _]
                            tunnel: w523 -> [w526 _]
                            tunnel: w522 -> [w529 _]
                            tunnel: w521 -> [w527 _]
                            tunnel: w520 -> [w528 _]
                            tunnel: [w525 _] -> w519
                            frame #0 {
                              n257 = for {
                                tunnel: w530 -> [w548]
                                tunnel: w526 -> [w547]
                                tunnel: w527 -> [w539] mode=indexing
                                tunnel: w528 -> [w533] mode=indexing
                                shift-right: [w537] -> w525
                                shift-left: w529 -> [w532]
                                n258 = local read "All Variables"() -> (w536:string[])
                                n259 = local read "Param_Value"() -> (w534:dbl[])
                                n260 = local read "Param_IDs"() -> (w535:string[])
                                n261 = call "Event Assign Calculator.vi"("Assign Val"=w533, "Param_Value"=w534, "Param_IDs"=w535, "All Variables"=w536, "transposed array"=w532) -> ("y value"=w531:dbl)  [unwired: 6 in]
                                n262 = Index Array(array=w532, index (col)=w539) -> (element=w542:dbl[])  [unwired: 1 in]
                                n263 = Index Array(array=w542, index=1) -> (element=w541:dbl)
                                n264 = local read "Delay Val Tot"() -> (w546:dbl[])
                                n265 = local read "Event Idx"() -> (w545:i32)
                                n266 = Index Array(array=w546, index=w545) -> (element=w544:dbl)
                                n267 = Greater Or Equal?(x=w547, y=w544) -> (x >= y?=w549:bool)
                                n268 = And(x=w548, y=w549) -> (x .and. y?=w550:bool)
                                n269 = Select(t=w531, s=w550, f=w541) -> (s? t:f=w538:dbl)
                                n270 = Replace Array Subset(array=w532, new element=w538, index (row)=1, index (col)=w539) -> (w537:dbl[][])
                              }
                            }
                            frame #1 {
                              n271 = local read "Del Events"() -> (w551:bool)
                              n272 = case shown="True" w551 {
                                frame False {
                                }
                                frame True {
                                n273 = local read "Assign Val"() -> (w556:string[][])
                                n274 = local read "Event Idx"() -> (w563:i32)
                                n275 = local read "Math Op"() -> (w562:string[])
                                n276 = local read "Math Val"() -> (w561:string[])
                                n277 = local read "Var Idx"() -> (w560:i32[])
                                n278 = Delete From Array(array=w561, length=1, index=w563) -> (array with subset deleted=w558:string[])  [unwired: 1 out]
                                n279 = Delete From Array(array=w560, length=1, index=w563) -> (array with subset deleted=w557:i32[])  [unwired: 1 out]
                                n280 = Delete From Array(array=w562, length=1, index=w563) -> (array with subset deleted=w559:string[])  [unwired: 1 out]
                                n281 = Delete From Array(array=w556, index (row)=w563) -> (array with subset deleted=w555:string[][])  [unwired: 2 in, 1 out]
                                n282 = local write "Assign Val"(w555) -> ()
                                n283 = local write "Math Op"(w559) -> ()
                                n284 = local write "Math Val"(w558) -> ()
                                n285 = local write "Var Idx"(w557) -> ()
                                n286 = local read "Assign Var Idx"() -> (w554:i32[][])
                                n287 = local read "Event Idx"() -> (w553:i32)
                                n288 = Delete From Array(array=w554, index (row)=w553) -> (array with subset deleted=w552:i32[][])  [unwired: 2 in, 1 out]
                                n289 = local write "Assign Var Idx"(w552) -> ()
                                }
                              }
                            }
                          }
                        }
                      }
                    }
                  }
                }
              }
            }
          }
          n290 = global read "Stop ODE.vi" "Stop ODE"() -> (w171:bool)
          "Event Idx" <- w170
        }
      }
      frame Disabled {
        n291 = local read "Delay Val Tot"() -> (w569:dbl[])
        n292 = local read "Delay"() -> (w571:dbl[])
        n293 = local read "Flag"() -> (w570:i32[])
        n294 = local read "Delay Val"() -> (w572:dbl)
        n295 = local read "Priority"() -> (w573:dbl[])
        n296 = call "SBML Events Handler.vi"("Sim Data w/ time"=w581, "Math Op"=w576, "Math Val"=w577, "Var Idx"=w578, "Idx of Time"=w579, "Assign Val"=w575, "Delay"=w571, "Assign Var Idx"=w574, "Flag"=w570, "Priority"=w573, "Delay Val Tot"=w569, "Delay Val"=w572) -> ("Output Data"=w580:dbl[][], "Flag Out"=w568:i32[], "Delay Val Tot Out"=w567:dbl[])  [unwired: 5 in]
        n297 = local write "Delay Val Tot"(w567) -> ()
        n298 = local write "Flag"(w568) -> ()
      }
    }
    "Array" <- w66
    n299 = global read "Stop ODE.vi" "Stop ODE"() -> (w91:bool)
    n300 = Array Subset(array=w66, index (col)=1 ("index (row)")) -> (w95:dbl[][])  [unwired: 3 in]
    "subarray" <- w95
    n301 = Index Array(array=w103, index=0) -> (element=w64:i32)
    n302 = Index Array(array=w103, index=1) -> (element=w94:i32)
    n303 = Decrement(x=w64) -> (x-1=w65:i32)
    n304 = Array Subset(array=w95, index (row)=w65, length (row)=1 ("length"), index (col)=0 ("length"), length (col)=w94) -> (w112:dbl[][])
    n305 = Array Subset(array=w95, index (col)=w94, length (col)=w92) -> (w81:dbl[][])  [unwired: 2 in]
    n306 = Array Subset(array=w95, index (col)=w94) -> (w102:dbl[][])  [unwired: 3 in]
    n307 = Index Array(array=w112) -> (element=w67:dbl[])  [unwired: 2 in]
    "subarray 2" <- w67
    n308 = Index Array(array=w81, index (row)=1) -> (element=w80:dbl[])  [unwired: 1 in]
    n309 = Index Array(array=w102) -> (element=w101:dbl[])  [unwired: 2 in]
  }
  n310 = local read "Initial Conditions for  variables"() -> (w23:dbl[])
  n311 = Array Size(array=w12) -> (size(s)=w20:i32[])
  n312 = Decrement(x=w20) -> (x-1=w18:i32[])
  n313 = Array Size(array=w28) -> (size(s)=w26:i32)
  n314 = Decrement(x=w26) -> (x-1=w25:i32)
  n315 = Index Array(array=w18, index=0) -> (element=w16:i32)
  n316 = Delete From Array(array=w12, length=1, index (row)=w16) -> (array with subset deleted=w15:dbl[][])  [unwired: 1 in, 1 out]
  n317 = Delete From Array(array=w28, length=1, index=w25) -> (array with subset deleted=w21:dbl[])  [unwired: 1 out]
  n318 = Insert Into Array(array=w15, index (row)=0, new element=w23) -> (w11:dbl[][])  [unwired: 1 in]
  n319 = Insert Into Array(array=w13, index (col)=0 ("disabled index (col)"), new element=w11) -> (w10:dbl[][])  [unwired: 1 in]
  n320 = Transpose 2D Array(2D array=w10) -> (transposed array=w24:dbl[][])
  n321 = Bundle("Time"=w21, w10) -> (→"Sim Data":cluster{"Time":dbl[], dbl[][]})  [unwired: 1 in]
  n322 = for {
    tunnel: w21 -> [w583]
    tunnel: [w584] -> w5 mode=indexing
    tunnel: w24 -> [w582] mode=indexing
    n323 = Bundle("Time"=w583, w582) -> (w584:cluster{"Time":dbl[], dbl[]})  [unwired: 1 out]
  }
  "Concentration vs. Time" <- w5
  n324 = flat-sequence {
    tunnel: w5 -> [_]
    frame #0 {
      n325 = global write "Stop ODE.vi" "Stop ODE"(TRUE) -> ()
      n326 = global write "Sim status.vi" "Status"(0 ("Status")) -> ()
    }
  }
  "Mod_IDs Out" <- "Mod_IDs"
  "Rest_Sp_IDs Out" <- "Rest_Sp_IDs"
